vi "Waveform Unflatten.vi"(8 "error in (no error)":errorcluster, 10 "Data in in":T2[](array[typedef]), 11 "Flatten Data in":u8[](array[numeric])) -> (0 "error out":errorcluster, 2 "Data out":T2[](array[typedef]), 3 "Flatten Data out":u8[](array[numeric]), 5 "Header out":T1)   [LabVIEW 2021]
uses:
  typedef/Datatype Waveform.ctl
  typedef/FIFO Header.ctl
  Utilities/Add Error.vi
  dd5197f3-4275-40d4-b3d5-d48df1723d2d.vi/c28b0ead-42ad-4072-80a2-aca7f2bd7ce3.vi
  4057d038-64e5-404a-b8d2-8db20ad085cb.vi/c28b0ead-42ad-4072-80a2-aca7f2bd7ce3.vi
  <vilib>/CIF Foundation/CIF Utilities/Errors/Append Error Location.vi
  ChannelCommon.lvlib
  <vilib>/CIF Foundation/CIF Utilities/DataTypes/DataTypes_CIF_U.lvlib
  8980f996-a542-42f1-9c98-910966e77ad2.vi
  ce8ba92d-590f-4e46-8b1c-68dfd5c82777.vi
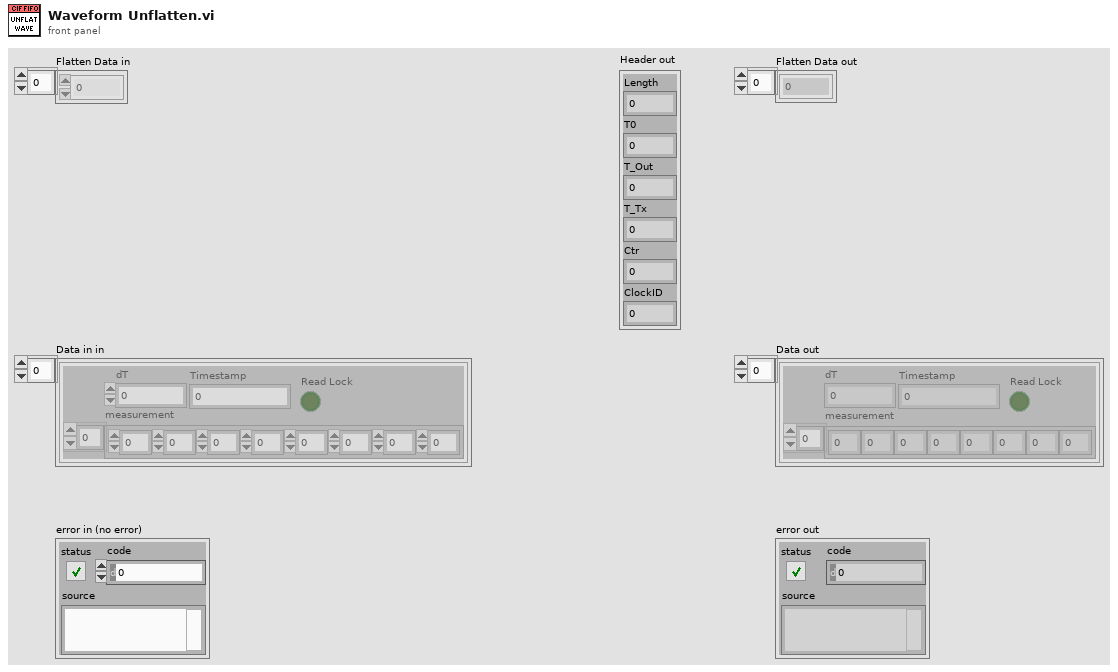
[diagram p1: front panel]
types:
  T1 = typedef "ChannelCommon.lvlib/FIFO Header.ctl" = cluster{"Length":u64, "T0":i64, "T_Out":i64, "T_Tx":i64, "Ctr":u64, "ClockID":u8}
  T2 = typedef "ChannelCommon.lvlib/Datatype Waveform.ctl" = cluster{"measurement":dbl[], "dT":dbl, "Timestamp":i64, "Read Lock":bool}
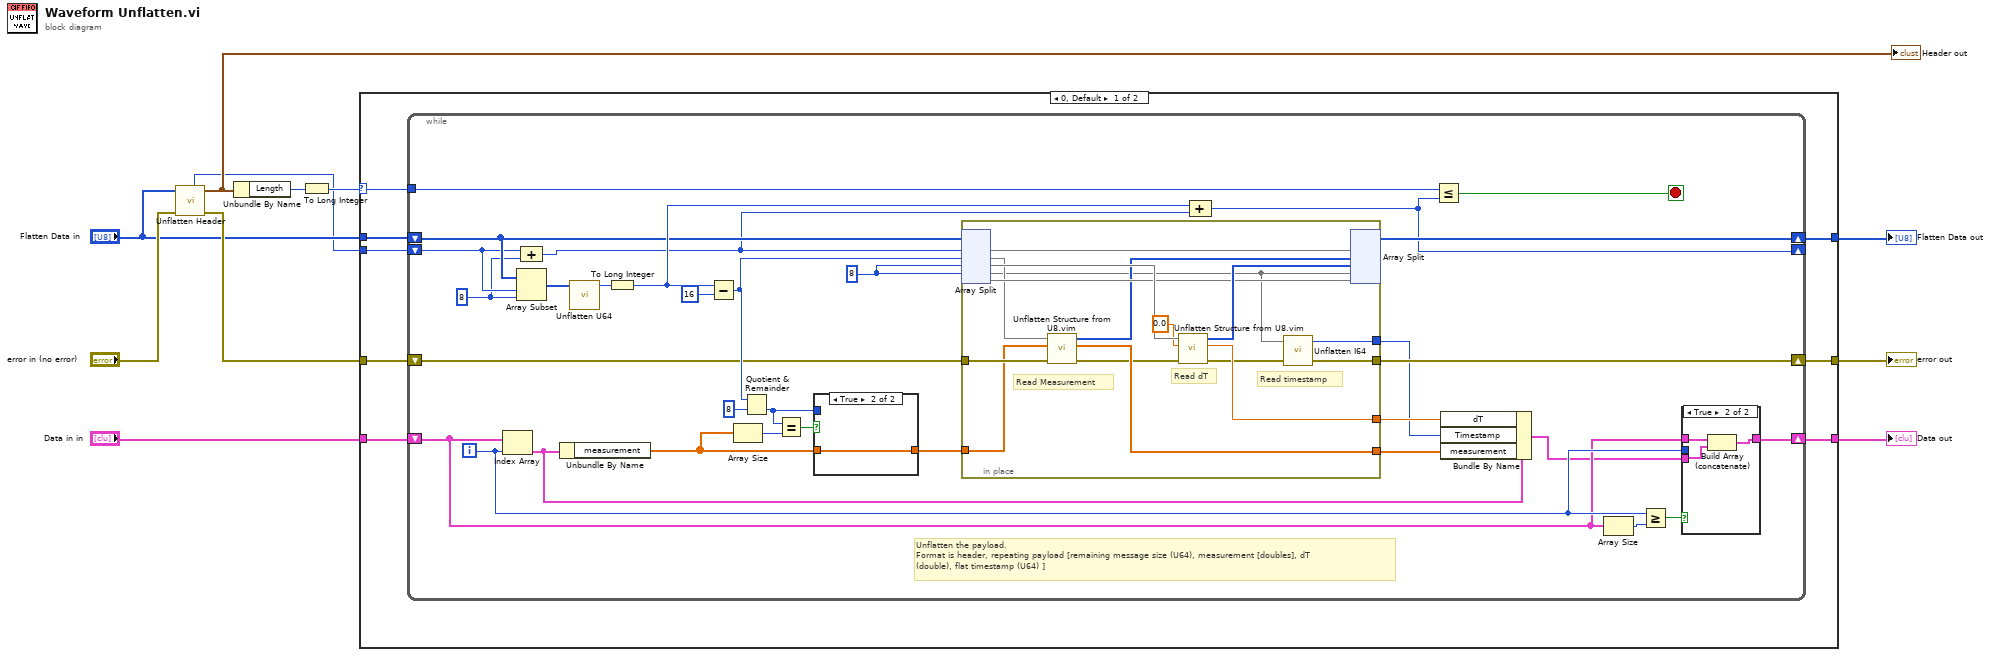
[diagram p0: block diagram]
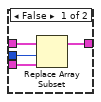
[diagram p2: hidden frame]
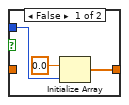
[diagram p3: hidden frame]
diagram:
  n1 = call "Unflatten Header.vi"("error in (no error)"="error in (no error)", "Flattened Data in"="Flatten Data in") -> ("error out"=w6:errorcluster, "Header out"=w4:T1, "offset out"=w1:i32)  [unwired: 7 in]
  "Header out" <- w4
  n2 = Unbundle By Name(w4) -> ("Length"=w5:u64)
  n3 = To Long Integer(number=w5) -> (32bit integer=w3:i32)
  n4 = case shown="0, Default" w3 {
    selector: w3 -> [w13 _]
    tunnel: [w19 w78] -> w11
    tunnel: "Data in in" -> [w18 w78]
    tunnel: [w17 w79] -> w9
    tunnel: [w16 w80] -> w8
    tunnel: "Flatten Data in" -> [w15 w80]
    tunnel: w6 -> [w14 w79]
    tunnel: w1 -> [w12 _]
    frame 0, Default {
      n5 = while {
        shift-right: [w50] -> w17
        shift-left: w14 -> [w21]
        shift-right: [w51] -> w16
        shift-left: w15 -> [w24]
        shift-right: [w48] -> _
        shift-left: w12 -> [w23]
        tunnel: w13 -> [w49]
        shift-right: [w46] -> w19
        shift-left: w18 -> [w30]
        i -> [w31]
        stop <- w47 stop-if-true
        w22 = 8 ("size")
        w40 = 8
        # "Unflatten the payload.\nFormat is header, repeating payload [remaining message size (U64), measurement [doubles], dT (double), flat timestamp (U64) ]"
        n6 = Index Array(array=w30, index=w31) -> (element=w45:T2)
        n7 = Array Subset(array=w24, index=w23, length=w22) -> (w27:u8[])
        n8 = Compound Arithmetic op=ADD(w23, w22) -> (w20:i32)
        n9 = Unbundle By Name(w45) -> ("measurement"=w34:dbl[])
        n10 = call <vilib>:"Unflatten U64.vi"("Flat Data"=w27) -> ("U64"=w26:u64)  [unwired: 4 in]
        n11 = To Long Integer(number=w26) -> (32bit integer=w25:i32)
        n12 = Subtract(x=w25, y=16) -> (x-y=w39:i32)
        n13 = Array Size(array=w34) -> (size(s)=w43:i32)
        n14 = Quotient & Remainder(x=w39, y=8) -> (floor(x/y)=w38:i32)  [unwired: 1 out]
        n15 = Equal?(x=w38, y=w43) -> (x = y?=w42:bool)
        n16 = case shown="True" w42 {
          tunnel: w34 -> [_ w62]
          tunnel: [w59 w62] -> w41
          tunnel: w38 -> [w61 _]
          frame False {
            n17 = Initialize Array(0.0, w61) -> (w59:dbl[])
          }
          frame True {
          }
        }
        n18 = in-place {
          in-place-border: [w68] -> w33
          in-place-border: [w73] -> w36
          in-place-border: [w64] -> w50
          in-place-border: w21 -> [w72]
          in-place-border: [w66] -> w35
          in-place-border: w41 -> [w69]
          # "Read timestamp"
          # "Read dT"
          # "Read Measurement"
          n19 = in-place-split #1(w24, w20, w39, w40, w40) -> (w77:u8[], w71:u8[], w76:u8[], w65:u8[], w74:u8[])
          n20 = call "Unflatten Structure from U8.vim"("error in"=w72, "Type"=w69, "Flattend Data in"=w71) -> ("error out"=w67:errorcluster, "Unflattend Data"=w68:dbl[], "Flatten Data out"=w70:u8[])  [unwired: 6 in]
          n21 = call "Unflatten Structure from U8.vim"("error in"=w67, "Type"=0.0, "Flattend Data in"=w76) -> ("error out"=w64:errorcluster, "Unflattend Data"=w73:dbl, "Flatten Data out"=w75:u8[])  [unwired: 6 in]
          n22 = call <vilib>:"Unflatten I64.vi"("Flat Data"=w65) -> ("I64"=w66:i64)  [unwired: 4 in]
          n23 = in-place-split #1(w77, w70, w75, w65, w74) -> (w51:u8[])  [unwired: 4 out]
        }
        n24 = Compound Arithmetic op=ADD(w25, w20) -> (w48:i32)
        n25 = Less Or Equal?(x=w49, y=w48) -> (x <= y?=w47:bool)
        n26 = Bundle By Name(cluster=w45, "dT"=w36, "Timestamp"=w35, "measurement"=w33) -> (w28:T2)
        n27 = Array Size(array=w30) -> (size(s)=w32:i32)
        n28 = Greater Or Equal?(x=w31, y=w32) -> (x >= y?=w29:bool)
        n29 = case shown="True" w29 {
          tunnel: w31 -> [w55 _]
          tunnel: w30 -> [w54 w58]
          tunnel: [w53 w56] -> w46
          tunnel: w28 -> [w52 w57]
          frame False {
            n30 = Replace Array Subset(array=w54, new element=w52, index=w55) -> (w53:T2[])
          }
          frame True {
            n31 = Build Array (concatenate)(w58, w57) -> (w56:T2[])
          }
        }
      }
    }
    frame 48 {
      # "Header only"
    }
  }
  "Data out" <- w11
  "error out" <- w9
  "Flatten Data out" <- w8
